vi "RSNRPZ Set Correction Frequency Spacing.vi"(8 "error in (no error)":errorcluster, 9 "Frequency Spacing (Linear)":i32(ring) items=["Linear", "Logarithmic"], 10 "Channel (1)":i32=1, 11 "VISA session":refnum<visa-resource-name> caption="VISA resource name") -> (0 "error out":errorcluster, 3 "dup VISA session":refnum<visa-resource-name> caption="VISA resource name")   [LabVIEW 2010]
doc: "If scalar network analysis is enabled this parameter defines how the frequency is incremented.\n\nLinear spacing means that the frequency step value is added to the current frequency after each buffered measurement.\nLogarithmic spacing means that the frequency step value is multiplied with the current frequency after each buffered measurement.\n\nThis command is used to do a simple scalar network nalysis. \nTo enable this automativally frequency stepping you have to configure CONTAV sensor mode, enable buffered measurements and set frequency stepping to a value greater than 0.\n\nRemote-control command(s):\nSENS:FREQ:SPAC"
uses:
  rsnrpz_32.dll
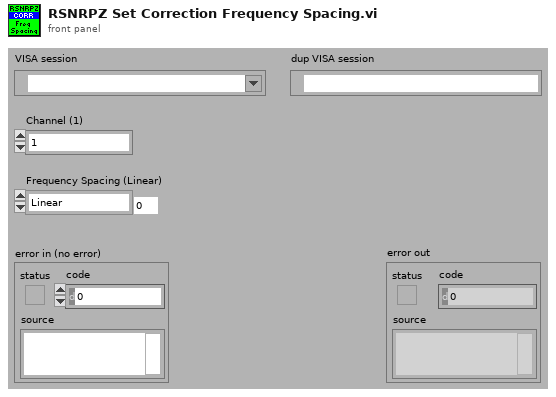
[diagram p1: front panel]
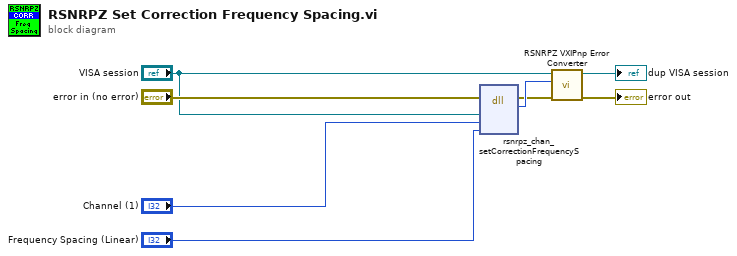
[diagram p0: block diagram]
diagram:
  n1 = dll-call lib="rsnrpz_32.dll" fn="rsnrpz_chan_setCorrectionFrequencySpacing"(error in="error in (no error)", "Instrument Handle"="VISA session", "Channel"="Channel (1)", "Frequency Spacing"="Frequency Spacing (Linear)") -> (error out=w5:errorcluster, w6:i32)  [unwired: 5 in, 1 out]
  n2 = call <instrlib>:"RSNRPZ VXIPnp Error Converter.vi"("error in"=w5, "VXIPnp error code"=w6, "VISA session"="VISA session") -> ("error out"=→"error out":errorcluster, "dup VISA session"=→"dup VISA session":refnum<visa-resource-name>)  [unwired: 7 in]
